vi "TL Motor MoveComplete.vi"() -> ()   [LabVIEW 2021]
panel:
  in  "stop":bool
  in  "MG17Motor":refnum<k7>(container)
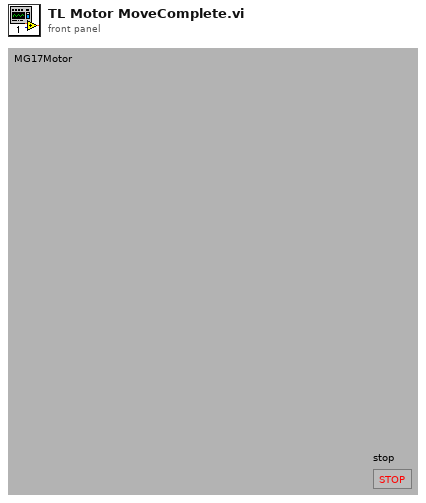
[diagram p1: front panel]
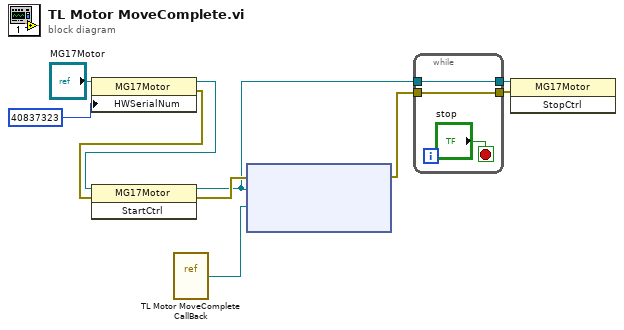
[diagram p0: block diagram]
diagram:
  n1 = property class="MG17Motor"(reference="MG17Motor", "HWSerialNum"=40837323) -> (reference out=w6:refnum<k7>, error out=w5:errorcluster)  [unwired: 1 in]
  n2 = invoke class="MG17Motor" method="StartCtrl"(reference=w6, error in=w5) -> (reference out=w2:refnum<k7>, error out=w8:errorcluster)  [unwired: 1 in, 1 out]
  n3 = vi-ref "TL Motor MoveComplete CallBack.vi"() -> ("vi reference"=w1:refnum<vi>)
  n4 = node(w8, w2, w1) -> (w7:errorcluster)  [unwired: 2 in, 1 out]
  n5 = while {
    tunnel: w7 -> [w12]
    tunnel: [w12] -> w4
    tunnel: [w11] -> w3
    tunnel: w2 -> [w11]
    stop <- "stop" stop-if-true
  }
  n6 = invoke class="MG17Motor" method="StopCtrl"(reference=w3, error in=w4) -> ()  [unwired: 1 in, 3 out]
